vi "231207_Webcam_Grab.vi"(8 "error in":errorcluster, 11 "Session In":T2="cam1") -> (0 "error out":errorcluster, 3 "Image":T1(plugin-control))   [LabVIEW 2023]
doc: "Vi qui permet d'afficher en live les images d'une caméra (webcam) et qui permet de sauver une image à un moment donné dans un fichier png"
uses:
  <vilib>/userDefined/High Color/IMAQdx.ctl
  <vilib>/vision/driver/NI_Vision_Acquisition_Software.lvlib
panel:
  in  "Full File Path":path
  in  "Menu":string(combo)="---"
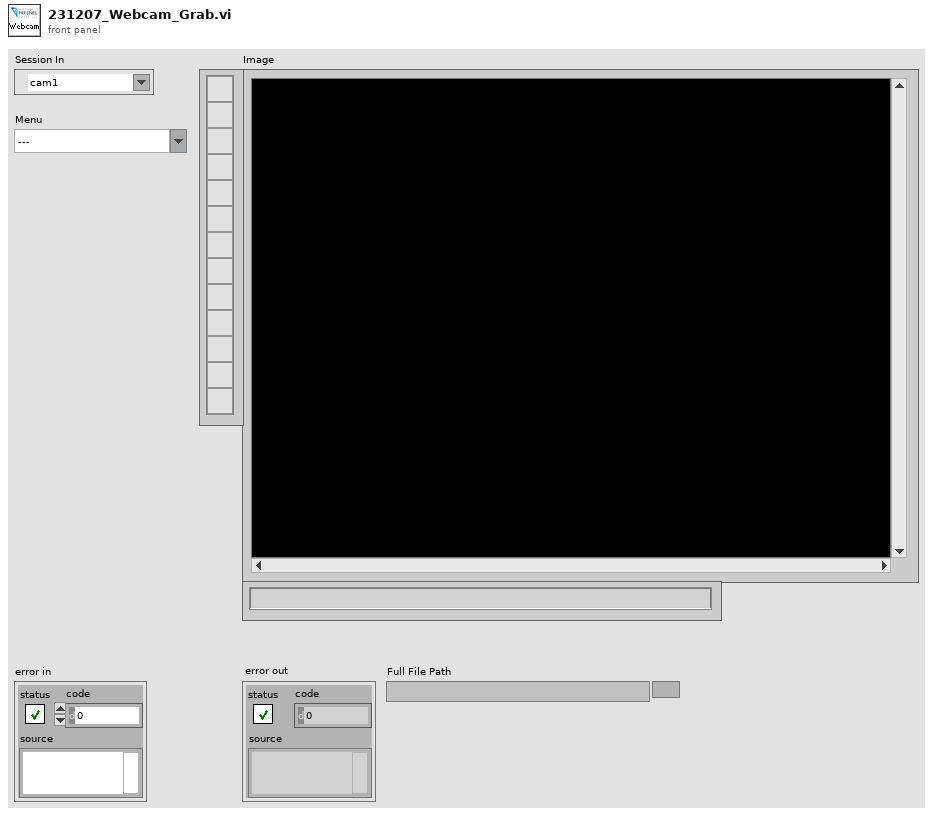
[diagram p1: front panel]
types:
  T1 = typedef "IMAQ Image.ctl" = refnum<image>
  T2 = typedef "IMAQdx.ctl" = refnum<k21>
  T3 = typedef "Image Type" = u32
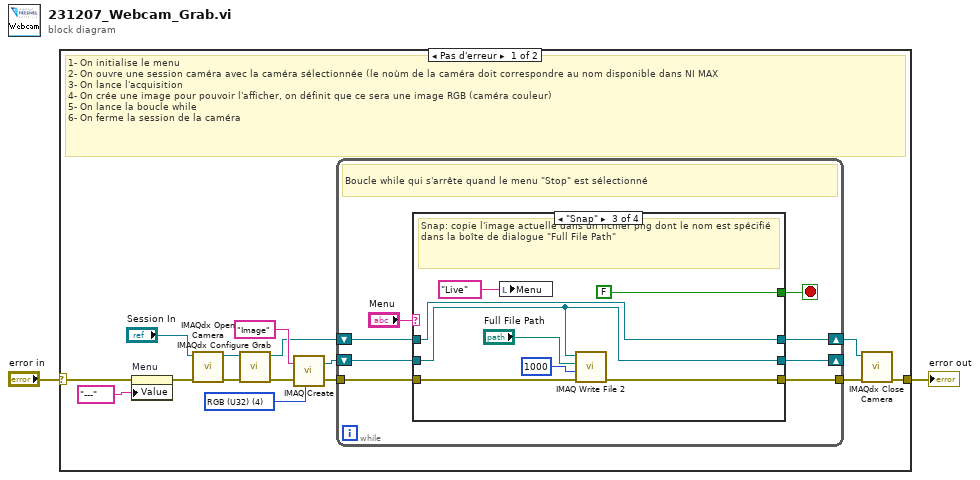
[diagram p0: block diagram]
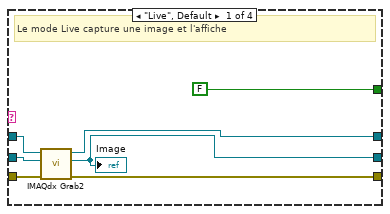
[diagram p2: hidden frame]
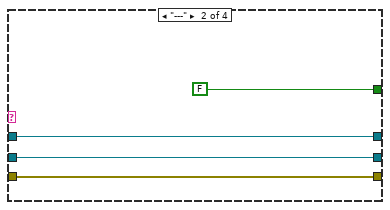
[diagram p3: hidden frame]
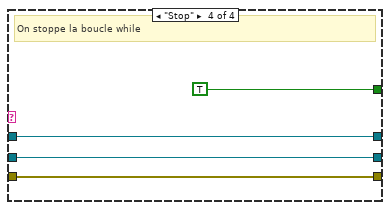
[diagram p4: hidden frame]
diagram:
  n1 = case shown="Pas d'erreur" "error in" {
    selector: "error in" -> [w5 w49]
    tunnel: [w11 w49] -> w2
    frame No Error {
      w12 = T3 4 items=["Grayscale (U8)", "Grayscale (I16)", "Grayscale (SGL)", "Complex (CSG)", "RGB (U32)", "HSL (U32)", "RGB (U64)", "Grayscale (U16)"] ("Image Type")
      # "1- On initialise le menu\n2- On ouvre une session caméra avec la caméra sélectionnée (le noùm de la caméra doit correspondre au nom disponible dans NI MAX\n3- On lance l'acquisition\n4- On crée une image pour pouvoir l'afficher, on définit que ce sera une image RGB (caméra couleur)\n5- On lance la boucle while\n6- On ferme la session de la caméra"
      n2 = property on="Menu" class="ChneDér"(error in=w5, "Value"="---" ("Menu")) -> (error out=w4:errorcluster)  [unwired: 1 in, 1 out]
      n3 = call <vilib>:"IMAQdx Open Camera.vi"("error in"=w4, "Session In"="Session In") -> ("error out"=w15:errorcluster, "Session Out"=w16:T2)  [unwired: 8 in]
      n4 = call <vilib>:"IMAQdx Configure Grab.vi"("error in"=w15, "Session In"=w16) -> ("error out"=w17:errorcluster, "Session Out"=w8:T2)  [unwired: 8 in]
      n5 = call "IMAQ Create"("Image Name"="Image", "Image Type"=w12, "error in (no error)"=w17) -> ("New Image"=w9:T1, "error out"=w10:errorcluster)  [unwired: 2 in]
      n6 = while {
        tunnel: w10 -> [w24]
        tunnel: [w23] -> w7
        shift-right: [w19] -> _
        shift-left: w9 -> [w20]
        shift-right: [w21] -> w6
        shift-left: w8 -> [w22]
        stop <- w25 stop-if-true
        # "Boucle while qui s'arrête quand le menu \"Stop\" est sélectionné"
        n7 = case shown="\"Snap\"" "Menu" {
          tunnel: [FALSE ("stop") FALSE ("stop") FALSE ("stop") TRUE ("stop")] -> w25
          tunnel: w24 -> [w31 w35 w41 w48]
          tunnel: [w30 w35 w40 w48] -> w23
          tunnel: w22 -> [w29 w33 w43 w46]
          tunnel: w20 -> [w28 w34 w42 w47]
          tunnel: [w27 w33 w43 w46] -> w21
          tunnel: [w26 w34 w42 w47] -> w19
          frame "Live", Default {
            # "Le mode Live capture une image et l'affiche"
            n8 = call <vilib>:"IMAQdx Grab2.vi"("error in"=w31, "Image In"=w28, "Session In"=w29) -> ("error out"=w30:errorcluster, "Image Out"=w26:T1, "Session Out"=w27:T2)  [unwired: 5 in, 1 out]
            "Image" <- w26
          }
          frame "---" {
          }
          frame "Snap" {
            # "Snap: copie l'image actuelle dans un fichier png dont le nom est spécifié dans la boîte de dialogue \"Full File Path\""
            n9 = local write "Menu"("Live" ("Menu")) -> ()
            n10 = call-poly "IMAQ Write File 2"("error in (no error)"=w41, "Image Quality"=u32 1000, "File Path"="Full File Path", "Image"=w42) -> ("error out"=w40:errorcluster)  [unwired: 6 in, 1 out]
          }
          frame "Stop" {
            # "On stoppe la boucle while"
          }
        }
      }
      n11 = call <vilib>:"IMAQdx Close Camera.vi"("error in"=w7, "Session In"=w6) -> ("error out"=w11:errorcluster)  [unwired: 9 in]
    }
    frame Error {
    }
  }
  "error out" <- w2
